vi "FRCts20_WebMethods_Team_PVT_bug.vi"(10 "team":string, 11 "httpRequestID":u32) -> ()   [LabVIEW 2014, in "FRCts20_WebMethods.lvlib"]
uses:
  FRCts20_WebMethods.lvlib
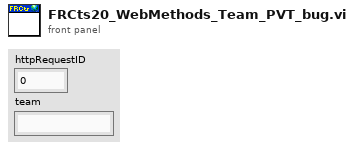
[diagram p1: front panel]
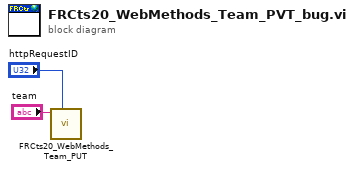
[diagram p0: block diagram]
diagram:
  n1 = call "FRCts20_WebMethods_Team_PUT.vi"("httpRequestID"="httpRequestID", "team"="team") -> ()  [unwired: 10 in]
